vi "Set 0(SubVI).vi"(8 "error in (no error)":errorcluster, 10 "Weak detect":bool, 11 "Control Cluster in":T1 {"Yaw Speed" scale=-1.0..1.0; "Vertical Speed" scale=-1.0..1.0; "Pitch" scale=-1.0..1.0; "Roll" scale=-1.0..1.0}) -> (0 "error out":errorcluster, 3 "Control Cluster out":T1 {"Yaw Speed" scale=-1.0..1.0; "Vertical Speed" scale=-1.0..1.0; "Pitch" scale=-1.0..1.0; "Roll" scale=-1.0..1.0})   [LabVIEW 2014]
uses:
  Resources/Others/Control cluster.ctl
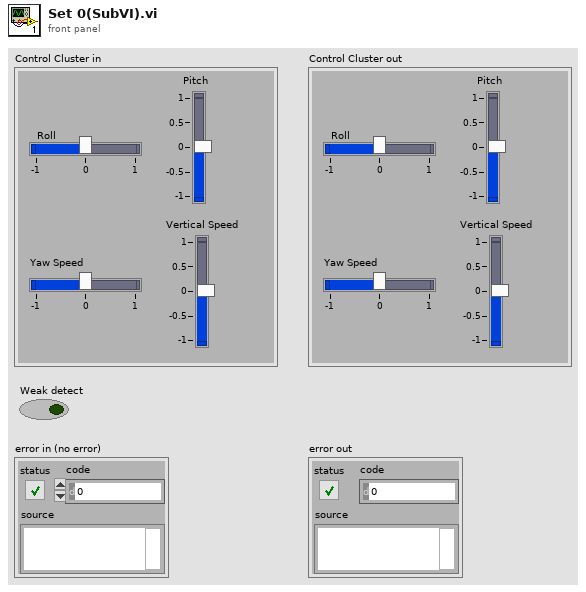
[diagram p1: front panel]
types:
  T1 = typedef "Control cluster.ctl" = cluster{"Roll":sgl, "Pitch":sgl, "Vertical Speed":sgl, "Yaw Speed":sgl}
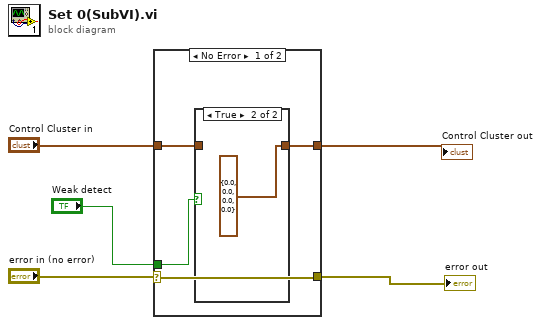
[diagram p0: block diagram]
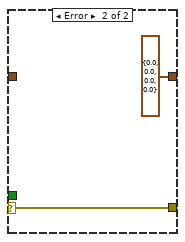
[diagram p3: hidden frame]
diagram:
  n1 = case shown="No Error" "error in (no error)" {
    selector: "error in (no error)" -> [w9 w12]
    tunnel: "Control Cluster in" -> [w7 _]
    tunnel: [w6 T1 {"Roll"=0.0, "Pitch"=0.0, "Vertical Speed"=0.0, "Yaw Speed"=0.0} ("Control Cluster out")] -> w3
    tunnel: [w9 w12] -> w4
    tunnel: "Weak detect" -> [w8 _]
    frame No Error {
      n2 = case shown="True" w8 {
        tunnel: w7 -> [w10 _]
        tunnel: [w10 T1 {"Roll"=0.0, "Pitch"=0.0, "Vertical Speed"=0.0, "Yaw Speed"=0.0} ("Control Cluster out")] -> w6
        frame False {
        }
        frame True {
        }
      }
    }
    frame Error {
    }
  }
  "error out" <- w4
  "Control Cluster out" <- w3
